vi "PMU_INFO.vi"(1 "data in":string) -> (0 "RET_DATA":T1)   [LabVIEW 2013]
panel:
  out "DIGUNIT":string
  out "ANUNIT":string
  out "PHUNIT":string
  out "DIGs":T2
  out "ANGs":T3
  out "PHASORS":T4
  out "NUMs":cluster{"PHNMR":u8, "ANNMR":u8, "DGNMR":u8}
  out "FORMAT":T5
  out "IDCODE":string
  out "Station Name":string
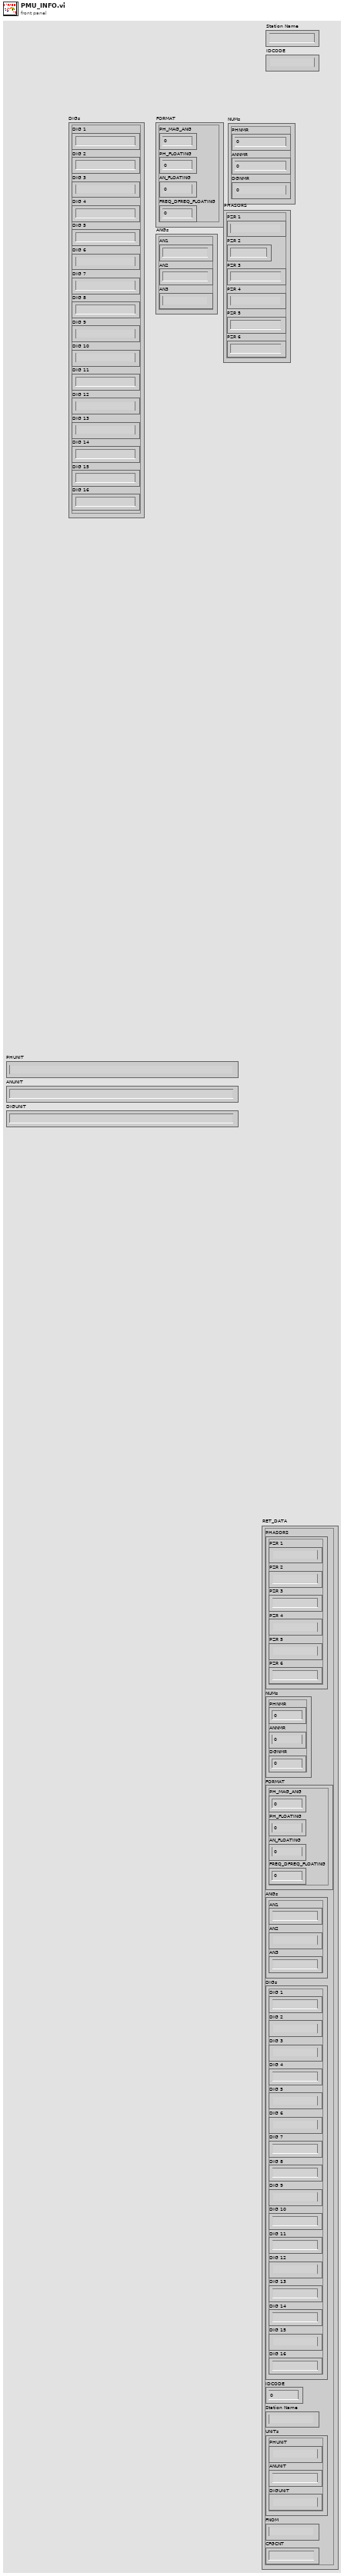
[diagram p1: front panel]
types:
  T1 = cluster{"PHASORS":cluster{"PZR 1":string, "PZR 2":string, "PZR 3":string, "PZR 4":string, "PZR 5":string, "PZR 6":string}, "NUMs":cluster{"PHNMR":u8, "ANNMR":u8, "DGNMR":u8}, "FORMAT":cluster{"PH_MAG_ANG":u16, "PH_FLOATING":u16, "AN_FLOATING":u16, "FREQ_DFREQ_FLOATING":u16}, "ANGs":cluster{"AN1":string, "AN2":string, "AN3":string}, "DIGs":cluster{"DIG 1":string, "DIG 2":string, "DIG 3":string, "DIG 4":string, "DIG 5":string, "DIG 6":string, "DIG 7":string, "DIG 8":string, "DIG 9":string, "DIG 10":string, "DIG 11":string, "DIG 12":string, "DIG 13":string, "DIG 14":string, "DIG 15":string, "DIG 16":string}, "IDCODE":u16, "Station Name":string, "UNITs":cluster{"PHUNIT":string, "ANUNIT":string, "DIGUNIT":string}, "FNOM":string, "CFGCNT":string}
  T2 = cluster{"DIG 1":string, "DIG 2":string, "DIG 3":string, "DIG 4":string, "DIG 5":string, "DIG 6":string, "DIG 7":string, "DIG 8":string, "DIG 9":string, "DIG 10":string, "DIG 11":string, "DIG 12":string, "DIG 13":string, "DIG 14":string, "DIG 15":string, "DIG 16":string}
  T3 = cluster{"AN1":string, "AN2":string, "AN3":string}
  T4 = cluster{"PZR 1":string, "PZR 2":string, "PZR 3":string, "PZR 4":string, "PZR 5":string, "PZR 6":string}
  T5 = cluster{"PH_MAG_ANG":u16, "PH_FLOATING":u16, "AN_FLOATING":u16, "FREQ_DFREQ_FLOATING":u16}
  T6 = cluster{"PHUNIT":string, "ANUNIT":string, "DIGUNIT":string}
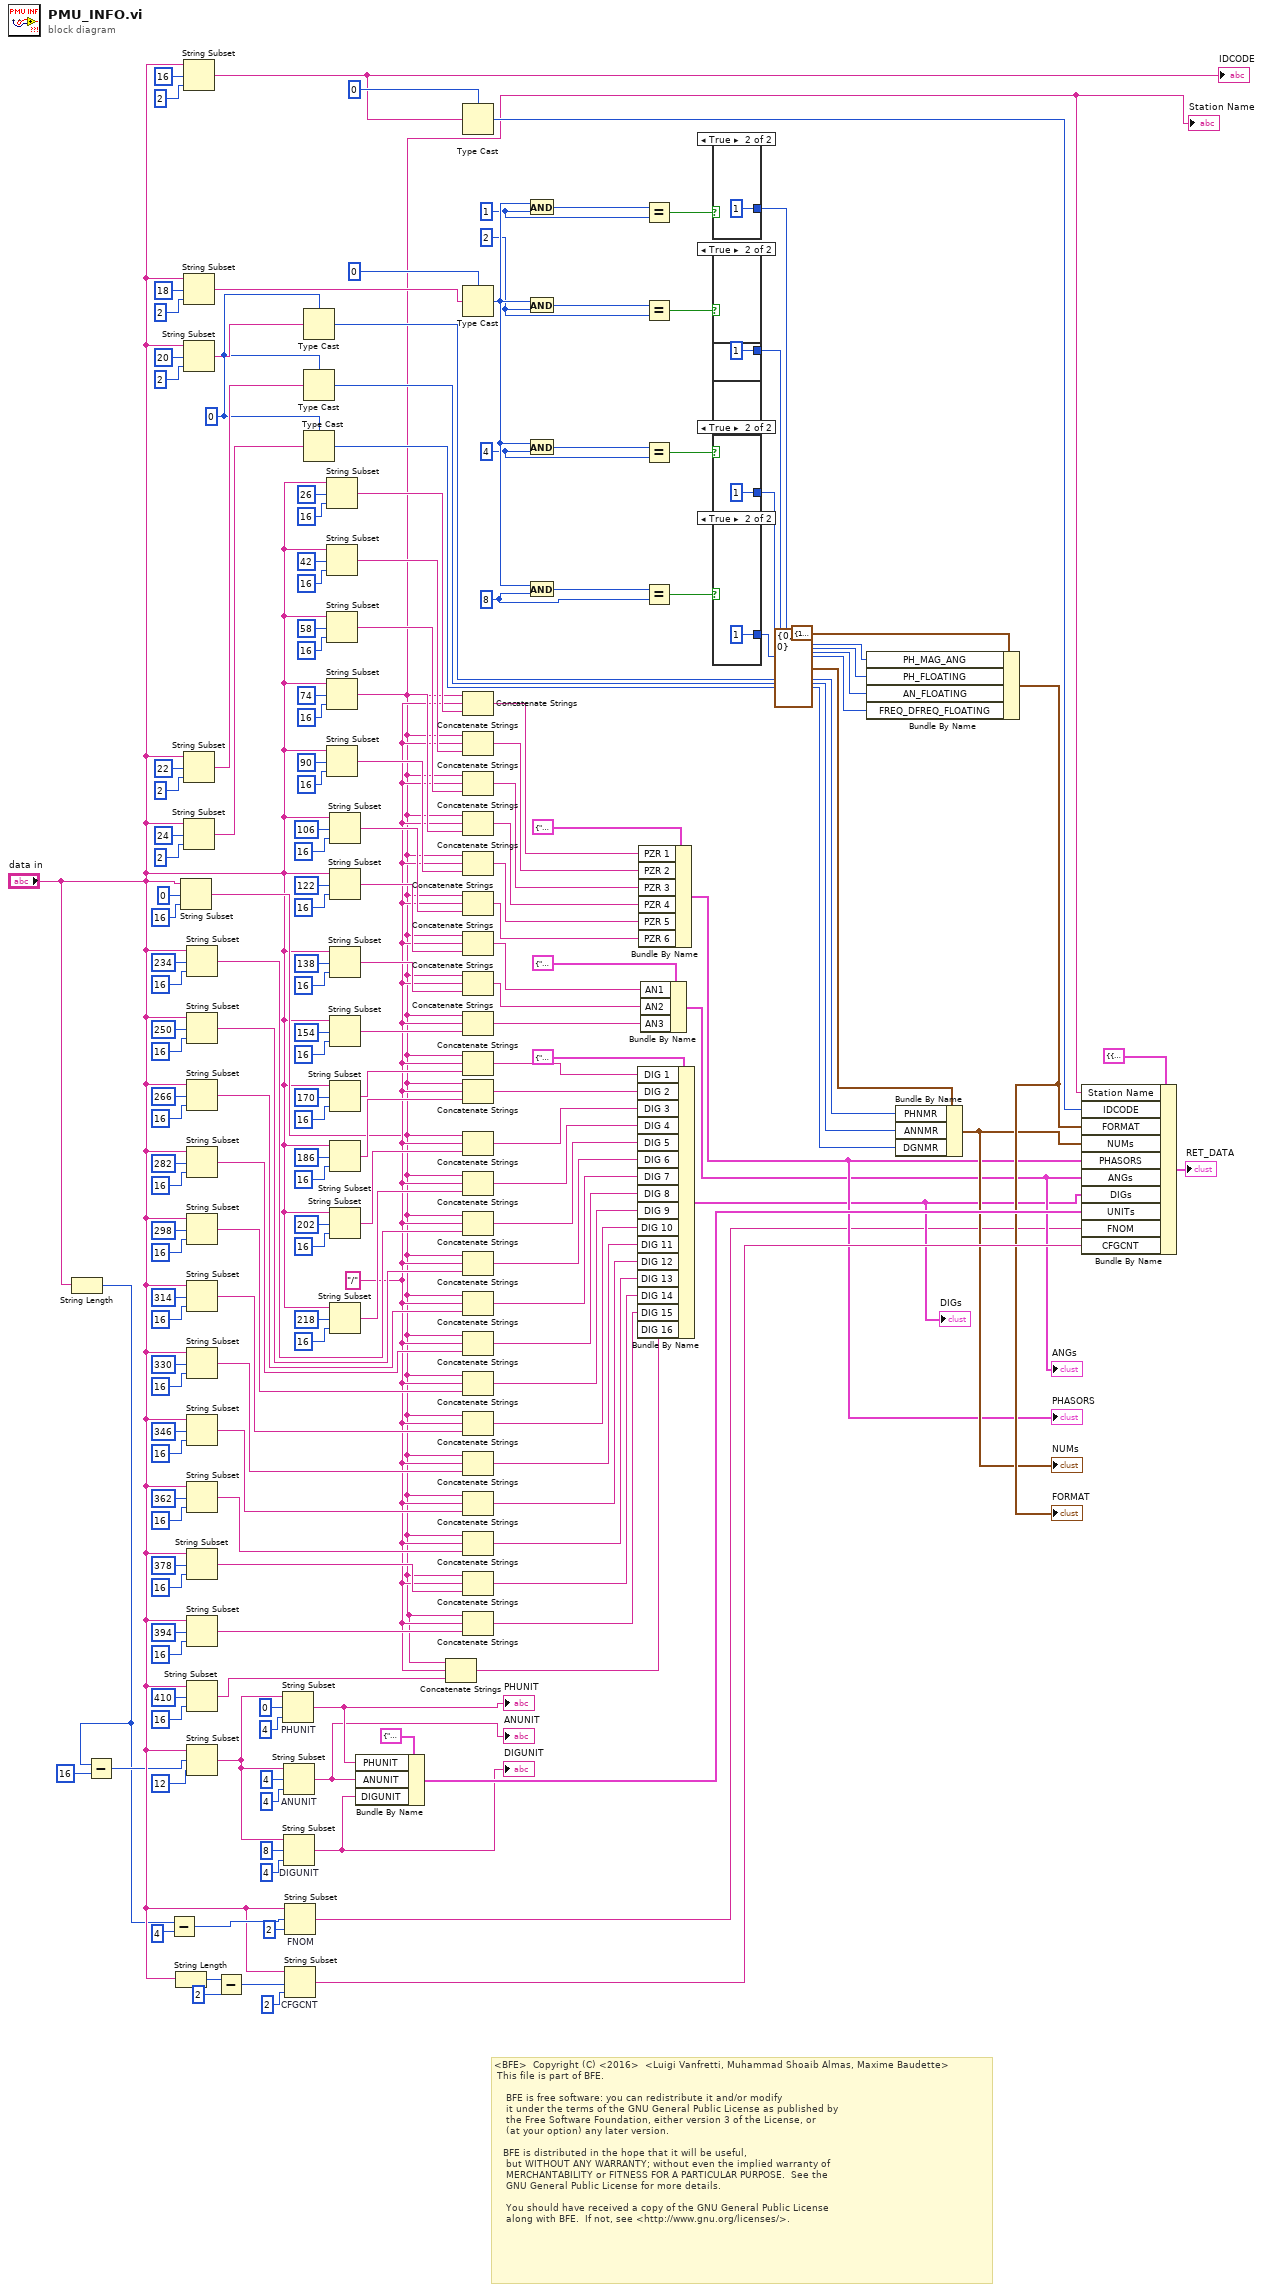
[diagram p0: block diagram]
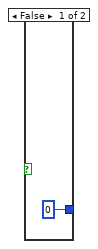
[diagram p2: hidden frame]
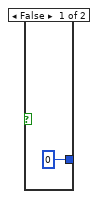
[diagram p3: hidden frame]
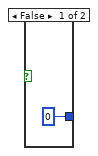
[diagram p4: hidden frame]
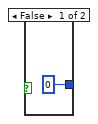
[diagram p5: hidden frame]
diagram:
  w20 = "/"
  w60 = u16 0
  w42 = u16 8 ("y")
  w46 = u16 4 ("y")
  w50 = u16 2 ("y")
  w54 = u16 1 ("y")
  # "<BFE>  Copyright (C) <2016>  <Luigi Vanfretti, Muhammad Shoaib Almas, Maxime Baudette>\n This file is part of BFE.\n\n    BFE is free software: you can redistribute it and/or modify\n    it under the terms of the GNU General Public License as published by\n    the Free Software Foundation, either version 3 of the License, or\n    (at your option) any later version.\n\n   BFE is distributed in the hope that it will be useful,\n    but WITHOUT ANY WARRANTY; without even the implied warranty of\n    MERCHANTABILITY or FITNESS FOR A PARTICULAR PURPOSE.  See the\n    GNU General Public License for more details.\n\n    You should have received a copy of the GNU General Public License\n    along with BFE.  If not, see <http://www.gnu.org/licenses/>."
  n1 = String Length(string="data in") -> (length=w2:i32)
  n2 = Subtract(x=w2, y=16) -> (x-y=w3:i32)
  n3 = Subtract(x=w2, y=4) -> (x-y=w7:i32)
  n4 = String Length(string="data in") -> (length=w11:i32)
  n5 = String Subset(string="data in", offset (0)=0, length (rest)=16 ("length (rest)")) -> (substring=w19:string)
  "Station Name" <- w19
  n6 = String Subset(string="data in", offset (0)=16, length (rest)=2 ("length (rest)")) -> (substring=w57:string)
  "IDCODE" <- w57
  n7 = String Subset(string="data in", offset (0)=18, length (rest)=2 ("length (rest)")) -> (substring=w171:string)
  n8 = String Subset(string="data in", offset (0)=20, length (rest)=2 ("length (rest)")) -> (substring=w166:string)
  n9 = String Subset(string="data in", offset (0)=22, length (rest)=2 ("length (rest)")) -> (substring=w165:string)
  n10 = String Subset(string="data in", offset (0)=24, length (rest)=2 ("length (rest)")) -> (substring=w163:string)
  n11 = String Subset(string="data in", offset (0)=234, length (rest)=16 ("length (rest)")) -> (substring=w97:string)
  n12 = String Subset(string="data in", offset (0)=250, length (rest)=16 ("length (rest)")) -> (substring=w98:string)
  n13 = String Subset(string="data in", offset (0)=266, length (rest)=16 ("length (rest)")) -> (substring=w99:string)
  n14 = String Subset(string="data in", offset (0)=282, length (rest)=16 ("length (rest)")) -> (substring=w100:string)
  n15 = String Subset(string="data in", offset (0)=298, length (rest)=16 ("length (rest)")) -> (substring=w101:string)
  n16 = String Subset(string="data in", offset (0)=314, length (rest)=16 ("length (rest)")) -> (substring=w102:string)
  n17 = String Subset(string="data in", offset (0)=330, length (rest)=16 ("length (rest)")) -> (substring=w103:string)
  n18 = String Subset(string="data in", offset (0)=346, length (rest)=16 ("length (rest)")) -> (substring=w104:string)
  n19 = String Subset(string="data in", offset (0)=362, length (rest)=16 ("length (rest)")) -> (substring=w105:string)
  n20 = String Subset(string="data in", offset (0)=378, length (rest)=16 ("length (rest)")) -> (substring=w106:string)
  n21 = String Subset(string="data in", offset (0)=394, length (rest)=16 ("length (rest)")) -> (substring=w37:string)
  n22 = String Subset(string="data in", offset (0)=410, length (rest)=16 ("length (rest)")) -> (substring=w21:string)
  n23 = String Subset(string="data in", offset (0)=w3, length (rest)=12 ("length (rest)")) -> (substring=w25:string)
  n24 = Subtract(x=w11, y=2) -> (x-y=w10:i32)
  n25 = String Subset "PHUNIT"(string=w25, offset (0)=0, length (rest)=4 ("length (rest)")) -> (substring=w24:string)
  "PHUNIT" <- w24
  n26 = String Subset "ANUNIT"(string=w25, offset (0)=4, length (rest)=4 ("length (rest)")) -> (substring=w22:string)
  "ANUNIT" <- w22
  n27 = String Subset "DIGUNIT"(string=w25, offset (0)=8, length (rest)=4 ("length (rest)")) -> (substring=w23:string)
  "DIGUNIT" <- w23
  n28 = String Subset "FNOM"(string="data in", offset (0)=w7, length (rest)=2 ("length (rest)")) -> (substring=w8:string)
  n29 = String Subset "CFGCNT"(string="data in", offset (0)=w10, length (rest)=2 ("length (rest)")) -> (substring=w27:string)
  n30 = Type Cast(type=w60, x=w166) -> (*(type *) &x=w65:u16)
  n31 = Type Cast(type=w60, x=w165) -> (*(type *) &x=w64:u16)
  n32 = Type Cast(type=w60, x=w163) -> (*(type *) &x=w63:u16)
  n33 = String Subset(string="data in", offset (0)=26, length (rest)=16 ("length (rest)")) -> (substring=w151:string)
  n34 = String Subset(string="data in", offset (0)=42, length (rest)=16 ("length (rest)")) -> (substring=w150:string)
  n35 = String Subset(string="data in", offset (0)=58, length (rest)=16 ("length (rest)")) -> (substring=w149:string)
  n36 = String Subset(string="data in", offset (0)=74, length (rest)=16 ("length (rest)")) -> (substring=w148:string)
  n37 = String Subset(string="data in", offset (0)=90, length (rest)=16 ("length (rest)")) -> (substring=w147:string)
  n38 = String Subset(string="data in", offset (0)=106, length (rest)=16 ("length (rest)")) -> (substring=w146:string)
  n39 = String Subset(string="data in", offset (0)=122, length (rest)=16 ("length (rest)")) -> (substring=w139:string)
  n40 = String Subset(string="data in", offset (0)=138, length (rest)=16 ("length (rest)")) -> (substring=w138:string)
  n41 = String Subset(string="data in", offset (0)=154, length (rest)=16 ("length (rest)")) -> (substring=w137:string)
  n42 = String Subset(string="data in", offset (0)=170, length (rest)=16 ("length (rest)")) -> (substring=w93:string)
  n43 = String Subset(string="data in", offset (0)=186, length (rest)=16 ("length (rest)")) -> (substring=w94:string)
  n44 = String Subset(string="data in", offset (0)=202, length (rest)=16 ("length (rest)")) -> (substring=w95:string)
  n45 = String Subset(string="data in", offset (0)=218, length (rest)=16 ("length (rest)")) -> (substring=w96:string)
  n46 = Bundle By Name(cluster=T6 {"PHUNIT"="", "ANUNIT"="", "DIGUNIT"=""}, "PHUNIT"=w24, "ANUNIT"=w22, "DIGUNIT"=w23) -> (w28:T6)
  n47 = Concatenate Strings(w19, w20, w21) -> (w18:string)
  n48 = Type Cast(type=u16 0, x=w57) -> (*(type *) &x=w56:u16)
  n49 = Type Cast(type=u16 0, x=w171) -> (*(type *) &x=w174:u16)
  n50 = Concatenate Strings(w19, w20, w151) -> (w76:string)
  n51 = Concatenate Strings(w19, w20, w150) -> (w75:string)
  n52 = Concatenate Strings(w19, w20, w149) -> (w74:string)
  n53 = Concatenate Strings(w19, w20, w148) -> (w73:string)
  n54 = Concatenate Strings(w19, w20, w147) -> (w72:string)
  n55 = Concatenate Strings(w19, w20, w146) -> (w71:string)
  n56 = Concatenate Strings(w19, w20, w139) -> (w69:string)
  n57 = Concatenate Strings(w19, w20, w138) -> (w68:string)
  n58 = Concatenate Strings(w19, w20, w137) -> (w67:string)
  n59 = Concatenate Strings(w19, w20, w93) -> (w92:string)
  n60 = Concatenate Strings(w19, w20, w94) -> (w91:string)
  n61 = Concatenate Strings(w19, w20, w95) -> (w90:string)
  n62 = Concatenate Strings(w19, w20, w96) -> (w79:string)
  n63 = Concatenate Strings(w19, w20, w97) -> (w89:string)
  n64 = Concatenate Strings(w19, w20, w98) -> (w88:string)
  n65 = Concatenate Strings(w19, w20, w99) -> (w78:string)
  n66 = Concatenate Strings(w19, w20, w100) -> (w87:string)
  n67 = Concatenate Strings(w19, w20, w101) -> (w86:string)
  n68 = Concatenate Strings(w19, w20, w102) -> (w85:string)
  n69 = Concatenate Strings(w19, w20, w103) -> (w84:string)
  n70 = Concatenate Strings(w19, w20, w104) -> (w83:string)
  n71 = Concatenate Strings(w19, w20, w105) -> (w82:string)
  n72 = Concatenate Strings(w19, w20, w106) -> (w81:string)
  n73 = Concatenate Strings(w19, w20, w37) -> (w80:string)
  n74 = And(x=w174, y=w54) -> (x .and. y?=w53:u16)
  n75 = And(x=w174, y=w50) -> (x .and. y?=w49:u16)
  n76 = And(x=w174, y=w46) -> (x .and. y?=w45:u16)
  n77 = And(x=w174, y=w42) -> (x .and. y?=w41:u16)
  n78 = Bundle By Name(cluster=T2 {"DIG 1"="PMU.133/DIG.stat1_01    ", "DIG 2"="PMU.133/DIG.stat1_02    ", "DIG 3"="PMU.133/DIG.stat1_03    ", "DIG 4"="PMU.133/DIG.stat1_04    ", "DIG 5"="PMU.133/DIG.stat1_05    ", "DIG 6"="PMU.133/DIG.stat1_06    ", "DIG 7"="PMU.133/DIG.stat1_07    ", "DIG 8"="PMU.133/DIG.stat1_08    ", "DIG 9"="PMU.133/DIG.stat1_09    ", "DIG 10"="PMU.133/DIG.stat1_10    ", "DIG 11"="PMU.133/DIG.stat1_11    ", "DIG 12"="PMU.133/DIG.stat1_12    ", "DIG 13"="PMU.133/DIG.stat1_13    ", "DIG 14"="PMU.133/DIG.stat1_14    ", "DIG 15"="PMU.133/DIG.stat1_15    ", "DIG 16"="PMU.133/DIG.stat1_15    "}, "DIG 1"=w92, "DIG 2"=w91, "DIG 3"=w90, "DIG 4"=w79, "DIG 5"=w89, "DIG 6"=w88, "DIG 7"=w78, "DIG 8"=w87, "DIG 9"=w86, "DIG 10"=w85, "DIG 11"=w84, "DIG 12"=w83, "DIG 13"=w82, "DIG 14"=w81, "DIG 15"=w80, "DIG 16"=w18) -> (w13:T2)
  "DIGs" <- w13
  n79 = Bundle By Name(cluster=T4 {"PZR 1"="PMU.133/PZR.AI          ", "PZR 2"="PMU.133/PZR.BV          ", "PZR 3"="PMU.133/PZR.CI          ", "PZR 4"="PMU.133/PZR.AV          ", "PZR 5"="PMU.133/PZR.BI          ", "PZR 6"="PMU.133/PZR.CV          "}, "PZR 1"=w76, "PZR 2"=w75, "PZR 3"=w74, "PZR 4"=w73, "PZR 5"=w72, "PZR 6"=w71) -> (w15:T4)
  "PHASORS" <- w15
  n80 = Bundle By Name(cluster=T3 {"AN1"="PMU.133/ANA1            ", "AN2"="PMU.133/ANA2            ", "AN3"="PMU.133/ANA3            "}, "AN1"=w69, "AN2"=w68, "AN3"=w67) -> (w14:T3)
  "ANGs" <- w14
  n81 = Equal?(x=w53, y=w54) -> (x = y?=w55:bool)
  n82 = Equal?(x=w49, y=w50) -> (x = y?=w51:bool)
  n83 = Equal?(x=w45, y=w46) -> (x = y?=w47:bool)
  n84 = Equal?(x=w41, y=w42) -> (x = y?=w43:bool)
  n85 = case shown="True" w55 {
    tunnel: [u16 0 ("y") u16 1 ("y")] -> w52
    frame False {
    }
    frame True {
    }
  }
  n86 = case shown="True" w51 {
    tunnel: [u16 0 ("y") u16 1 ("y")] -> w48
    frame False {
    }
    frame True {
    }
  }
  n87 = case shown="True" w47 {
    tunnel: [u16 0 ("y") u16 1 ("y")] -> w44
    frame False {
    }
    frame True {
    }
  }
  n88 = case shown="True" w43 {
    tunnel: [u16 0 ("y") u16 1 ("y")] -> w40
    frame False {
    }
    frame True {
    }
  }
  n89 = Bundle By Name(cluster=T5 {"PH_MAG_ANG"=1, "PH_FLOATING"=2, "AN_FLOATING"=4, "FREQ_DFREQ_FLOATING"=8}, "PH_MAG_ANG"=w52, "PH_FLOATING"=w48, "AN_FLOATING"=w44, "FREQ_DFREQ_FLOATING"=w40) -> (w17:T5)
  "FORMAT" <- w17
  n90 = Bundle By Name(cluster=cluster{"PHNMR":u8, "ANNMR":u8, "DGNMR":u8} {"PHNMR"=0, "ANNMR"=0, "DGNMR"=0}, "PHNMR"=w65, "ANNMR"=w64, "DGNMR"=w63) -> (w16:cluster{"PHNMR":u8, "ANNMR":u8, "DGNMR":u8})
  "NUMs" <- w16
  n91 = Bundle By Name(cluster=T1 {"PHASORS"={"PZR 1"="PMU.133/PZR.AI          ", "PZR 2"="PMU.133/PZR.BV          ", "PZR 3"="PMU.133/PZR.CI          ", "PZR 4"="PMU.133/PZR.AV          ", "PZR 5"="PMU.133/PZR.BI          ", "PZR 6"="PMU.133/PZR.CV          "}, "NUMs"={"PHNMR"=6, "ANNMR"=3, "DGNMR"=1}, "FORMAT"={"PH_MAG_ANG"=1, "PH_FLOATING"=2, "AN_FLOATING"=4, "FREQ_DFREQ_FLOATING"=8}, "ANGs"={"AN1"="PMU.133/ANA1            ", "AN2"="PMU.133/ANA2            ", "AN3"="PMU.133/ANA3            "}, "DIGs"={"DIG 1"="PMU.133/DIG.stat1_01    ", "DIG 2"="PMU.133/DIG.stat1_02    ", "DIG 3"="PMU.133/DIG.stat1_03    ", "DIG 4"="PMU.133/DIG.stat1_04    ", "DIG 5"="PMU.133/DIG.stat1_05    ", "DIG 6"="PMU.133/DIG.stat1_06    ", "DIG 7"="PMU.133/DIG.stat1_07    ", "DIG 8"="PMU.133/DIG.stat1_08    ", "DIG 9"="PMU.133/DIG.stat1_09    ", "DIG 10"="PMU.133/DIG.stat1_10    ", "DIG 11"="PMU.133/DIG.stat1_11    ", "DIG 12"="PMU.133/DIG.stat1_12    ", "DIG 13"="PMU.133/DIG.stat1_13    ", "DIG 14"="PMU.133/DIG.stat1_14    ", "DIG 15"="PMU.133/DIG.stat1_15    ", "DIG 16"="PMU.133/DIG.stat1_15    "}, "IDCODE"=0, "Station Name"="PMU.133", "UNITs"={"PHUNIT"="", "ANUNIT"="", "DIGUNIT"=""}, "FNOM"="", "CFGCNT"=""}, "Station Name"=w19, "IDCODE"=w56, "FORMAT"=w17, "NUMs"=w16, "PHASORS"=w15, "ANGs"=w14, "DIGs"=w13, "UNITs"=w28, "FNOM"=w8, "CFGCNT"=w27) -> (→"RET_DATA":T1)
